vi "CurrentInput_rawspeed.vi"(8 "Mode":u16(ring) items=["Log w/ Exp Z", "Log w/ Lin Z"], 9 "Maximum (pA)":dbl=9000.0, 10 "Current (pA)":dbl format="%.1f", 11 "Setpoint (A)":dbl=100.0) -> (2 "Setpoint (pA)":dbl, 3 "Filtered Current (pA)":dbl format="%.1f", 7 "Safetip?":bool)   [LabVIEW 2017]
uses:
  Program Files/National Instruments/LabVIEW 2019/user.lib/HapticSTM/HapticSTM.lvlib
  <vilib>/ptbypt/NI_PtbyPt.lvlib
  <vilib>/Analysis/3filter.llb/Filter Passband Type.ctl
  <vilib>/Analysis/NI_AALBase.lvlib
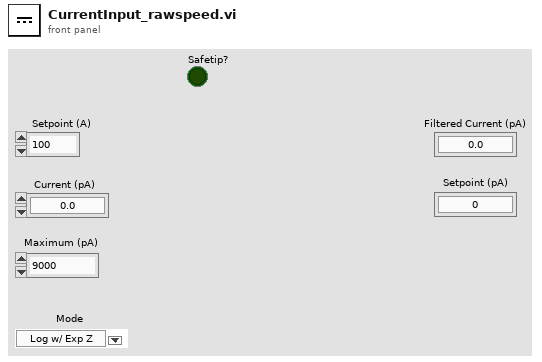
[diagram p1: front panel]
types:
  T1 = typedef "NI_AALBase.lvlib/Filter Passband Type.ctl" = enum32{"Lowpass", "Highpass", "Bandpass", "Bandstop"}
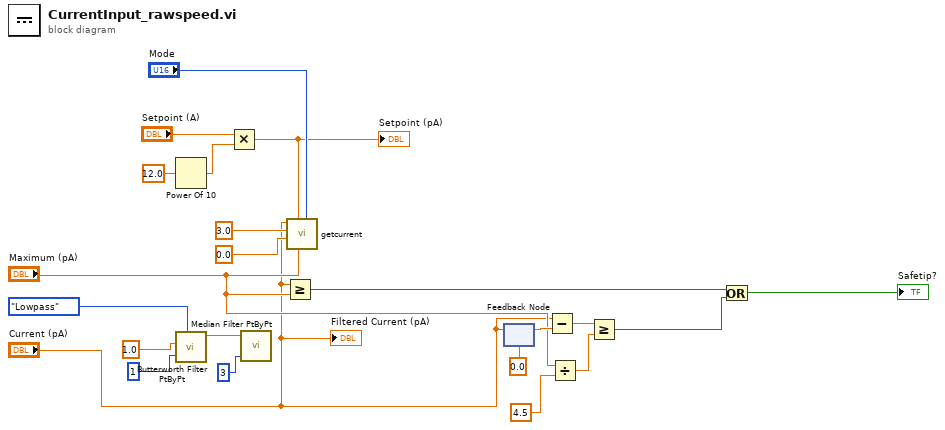
[diagram p0: block diagram]
diagram:
  n1 = Power Of 10(x=12.0) -> (10^x=w20:dbl)
  n2 = call <vilib>:"Butterworth Filter PtByPt.vi"("order"=1, "filter type"=Filter_Passband_Type."Lowpass", "sampling freq: fs"=1.0) -> ("Filtered x"=w15:dbl)  [unwired: 6 in, 1 out]
  n3 = Multiply(x="Setpoint (A)", y=w20) -> (x*y=w11:dbl)
  "Setpoint (pA)" <- w11
  n4 = call <vilib>:"Median Filter PtByPt.vi"("rank"=3, "x"=w15) -> ()  [unwired: 2 in, 2 out]
  n5 = Greater Or Equal?(x="Current (pA)", y="Maximum (pA)") -> (x >= y?=w12:bool)
  n6 = call "getcurrent.vi"("forcemode"="Mode", "maxcurrentin"="Maximum (pA)", "setpoint"=w11, "minforcey"=0.0, "maxforcey"=3.0, "currentin"="Current (pA)") -> ()  [unwired: 6 in]
  n7 = feedback-in #1("Current (pA)") -> ()
  n8 = feedback #1(0.0 ("Current (pA)")) -> (w8:dbl)
  n9 = Subtract(x="Current (pA)", y=w8) -> (x-y=w6:dbl)
  n10 = Divide(x="Maximum (pA)", y=4.5) -> (x/y=w4:dbl)
  n11 = Greater Or Equal?(x=w6, y=w4) -> (x >= y?=w5:bool)
  n12 = Or(x=w12, y=w5) -> (x .or. y?=→"Safetip?":bool)
  "Filtered Current (pA)" <- "Current (pA)"
